vi "JLINKARM Exec Command.vi"(8 "error in (no error)":errorcluster caption="错误输入（无错误）", 9 "param2":i32, 10 "param1":i32, 11 "pbCommand":string) -> (0 "error out":errorcluster caption="错误输出", 2 "function return":i32, 3 "pbCommand out":string)   [LabVIEW 2016, in "JLinkARM.lvlib"]
doc: "int JLINKARM_ExecCommand(char * pbCommand,int param1,int param2);"
uses:
  <userlib>/LV-JLinkARM/JLinkARM.lvlib
  <userlib>/LV-JLinkARM/JLinkARM.dll
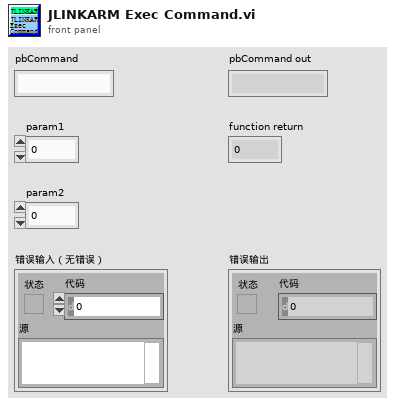
[diagram p1: front panel]
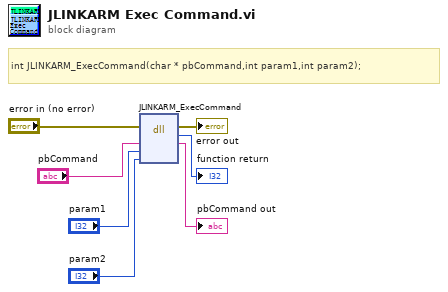
[diagram p0: block diagram]
diagram:
  # "int JLINKARM_ExecCommand(char * pbCommand,int param1,int param2);"
  n1 = dll-call lib="C:/Program Files (x86)/National Instruments/LabVIEW 2016/user.lib/LV-JLinkARM/JLinkARM.*" fn="JLINKARM_ExecCommand"(error in="error in (no error)", "pbCommand"="pbCommand", "param1"="param1", "param2"="param2") -> (error out=→"error out":errorcluster, →"function return":i32, "pbCommand"=→"pbCommand out":string)  [unwired: 4 in, 1 out]
